vi "External Interface - Find Control Reference.vi"(0 "Control References - Top Level":refnum<vi>[](array[refnum]), 7 "Control Name":string) -> (4 "Ctl Refnum":refnum<vi>, 8 "Found":bool, 15 "error out":errorcluster)   [LabVIEW 2010]
panel:
  out "Control Names":string[](array[string])
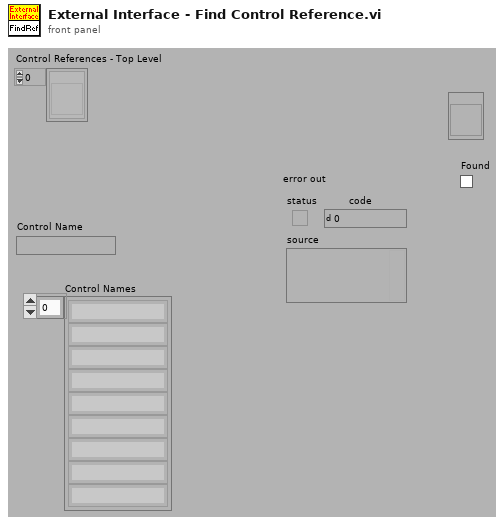
[diagram p1: front panel]
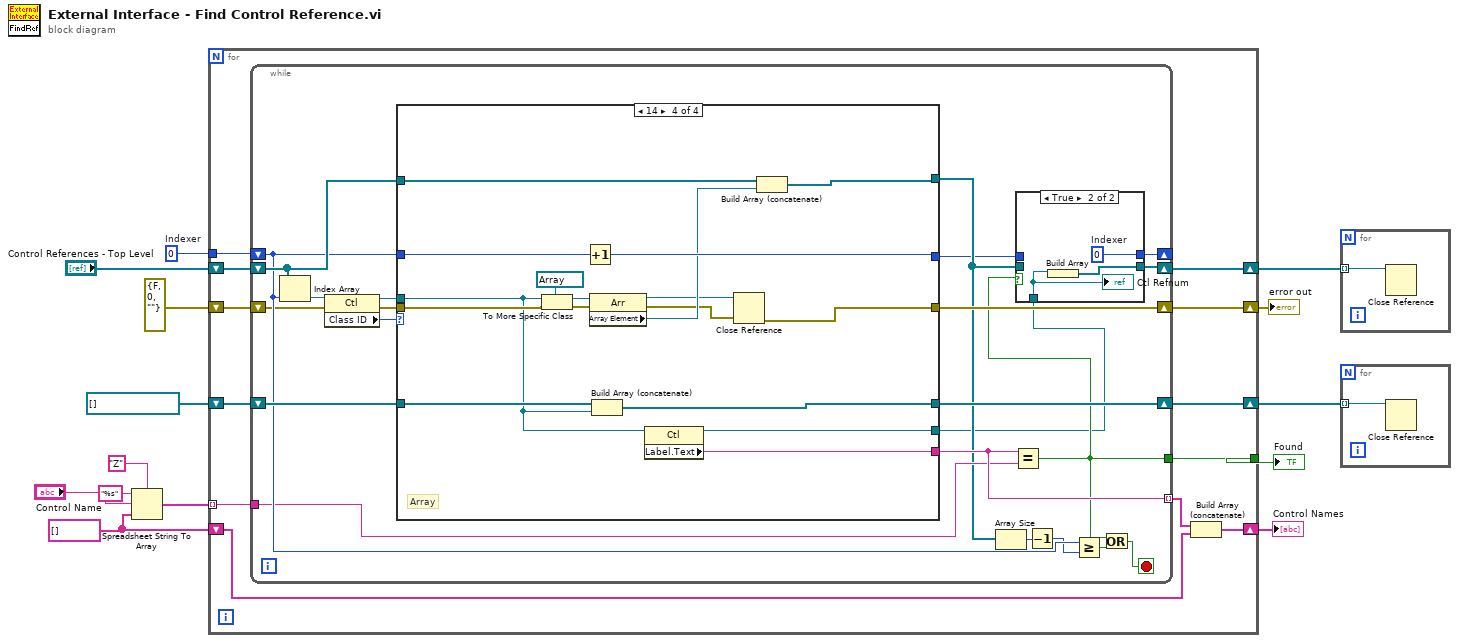
[diagram p0: block diagram]
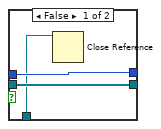
[diagram p2: hidden frame]
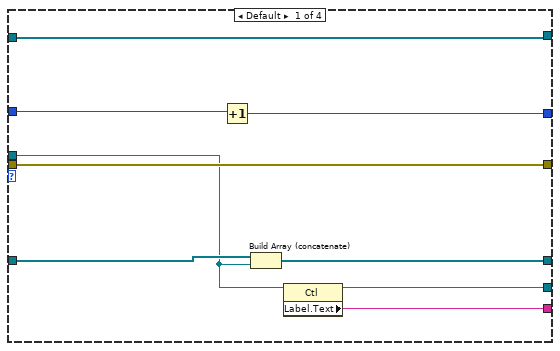
[diagram p3: hidden frame]
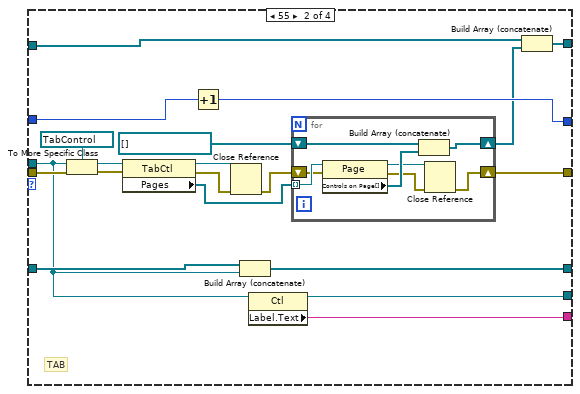
[diagram p4: hidden frame]
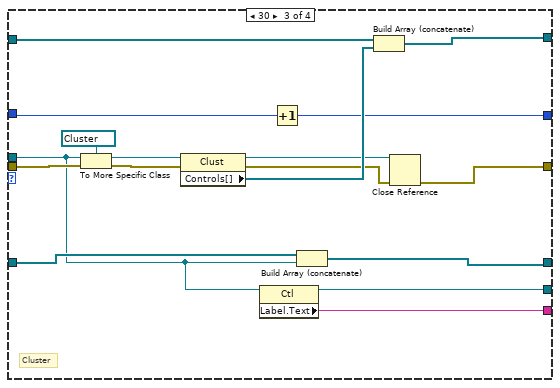
[diagram p5: hidden frame]
diagram:
  w4 = string[] []
  w13 = 0  # Indexer
  n1 = Spreadsheet String To Array(delimiter (Tab)="Ζ", format string="%s", spreadsheet string="Control Name", array type (2D Dbl)=w4) -> (array=w6:string[])
  n2 = for {
    tunnel: w13 -> [w25]
    tunnel: [w22] -> w10
    tunnel: w6 -> [w20] mode=indexing
    shift-right: [w24] -> w12
    shift-left: errorcluster {"status"=FALSE, "code"=0, "source"=""} ("error in") -> [w23]
    shift-right: [w21] -> w2
    shift-left: refnum<vi>[] [] -> [w26]
    shift-right: [w19] -> w1
    shift-left: "Control References - Top Level" -> [w18]
    shift-right: [w15] -> w3
    shift-left: w4 -> [w16]
    n3 = while {
      shift-right: [w46] -> w21
      shift-left: w26 -> [w47]
      shift-right: [w31] -> w19
      shift-left: w18 -> [w44]
      shift-right: [w30] -> _
      shift-left: w25 -> [w42]
      shift-right: [w40] -> w24
      shift-left: w23 -> [w41]
      tunnel: [w28] -> w22
      tunnel: [w34] -> w17 mode=indexing
      tunnel: w20 -> [w33]
      stop <- w35 stop-if-true
      n4 = Index Array(array=w44, index=w42) -> (element=w45:refnum<vi>)
      n5 = property class="Ctl"(reference=w45, error in=w41) -> (reference out=w48:refnum<vi>, error out=w39:errorcluster, "Class ID"=w37:u32)
      n6 = case shown="14" w37 {
        tunnel: w48 -> [w57 w70 w97 w114]
        tunnel: w47 -> [w58 w71 w101 w116]
        tunnel: [w63 w77 w102 w115] -> w46
        tunnel: [w62 w81 w108 w122] -> w32
        tunnel: w44 -> [w62 w79 w99 w123]
        tunnel: w42 -> [w61 w76 w100 w121]
        tunnel: [w60 w80 w98 w124] -> w29
        tunnel: w39 -> [w59 w74 w106 w119]
        tunnel: [w59 w72 w92 w109] -> w40
        tunnel: [w56 w69 w96 w113] -> w34
        tunnel: [w55 w68 w95 w112] -> w27
        frame Default {
          n7 = Increment(x=w61) -> (x+1=w60:i32)
          n8 = Build Array (concatenate)(w58, w57) -> (w63:refnum<vi>[])
          n9 = property class="Ctl"(reference=w57) -> (reference out=w55:refnum<vi>, "Label.Text"=w56:string)  [unwired: 1 in, 1 out]
        }
        frame 55 {
          # "TAB"
          n10 = To More Specific Class(target class=refnum<vi> refnum ("TabCtl Refnum"), reference=w70, error in=w74) -> (specific class reference=w83:refnum<vi>, error out=w73:errorcluster)
          n11 = property class="TabCtl"(reference=w83, error in=w73) -> (reference out=w66:refnum<vi>, error out=w65:errorcluster, "Pages"=w67:refnum<vi>[])
          n12 = Increment(x=w76) -> (x+1=w80:i32)
          n13 = Close Reference(reference=w66, error in (no error)=w65) -> (error out=w64:errorcluster)
          n14 = Build Array (concatenate)(w71, w70) -> (w77:refnum<vi>[])
          n15 = property class="Ctl"(reference=w70) -> (reference out=w68:refnum<vi>, "Label.Text"=w69:string)  [unwired: 1 in, 1 out]
          n16 = for {
            tunnel: w67 -> [w91] mode=indexing
            shift-right: [w89] -> w78
            shift-left: refnum<vi>[] [] -> [w90]
            shift-right: [w84] -> w72
            shift-left: w64 -> [w88]
            n17 = property class="Page"(reference=w91, error in=w88) -> (reference out=w86:refnum<vi>, error out=w85:errorcluster, "Controls on Page[]"=w87:refnum<vi>[])
            n18 = Build Array (concatenate)(w90, w87) -> (w89:refnum<vi>[])
            n19 = Close Reference(reference=w86, error in (no error)=w85) -> (error out=w84:errorcluster)
          }
          n20 = Build Array (concatenate)(w79, w78) -> (w81:refnum<vi>[])
        }
        frame 30 {
          # "Cluster"
          n21 = To More Specific Class(target class=refnum<vi> refnum ("Clust Refnum"), reference=w97, error in=w106) -> (specific class reference=w103:refnum<vi>, error out=w105:errorcluster)
          n22 = property class="Clust"(reference=w103, error in=w105) -> (reference out=w94:refnum<vi>, error out=w93:errorcluster, "Controls[]"=w104:refnum<vi>[])
          n23 = property class="Ctl"(reference=w97) -> (reference out=w95:refnum<vi>, "Label.Text"=w96:string)  [unwired: 1 in, 1 out]
          n24 = Increment(x=w100) -> (x+1=w98:i32)
          n25 = Build Array (concatenate)(w101, w97) -> (w102:refnum<vi>[])
          n26 = Build Array (concatenate)(w99, w104) -> (w108:refnum<vi>[])
          n27 = Close Reference(reference=w94, error in (no error)=w93) -> (error out=w92:errorcluster)
        }
        frame 14 {
          # "Array"
          n28 = To More Specific Class(target class=refnum<vi> refnum ("Array Refnum"), reference=w114, error in=w119) -> (specific class reference=w125:refnum<vi>, error out=w118:errorcluster)
          n29 = Increment(x=w121) -> (x+1=w124:i32)
          n30 = property class="Arr"(reference=w125, error in=w118) -> (reference out=w111:refnum<vi>, error out=w110:errorcluster, "Array Element"=w117:refnum<vi>)
          n31 = Build Array (concatenate)(w116, w114) -> (w115:refnum<vi>[])
          n32 = property class="Ctl"(reference=w114) -> (reference out=w112:refnum<vi>, "Label.Text"=w113:string)  [unwired: 1 in, 1 out]
          n33 = Close Reference(reference=w111, error in (no error)=w110) -> (error out=w109:errorcluster)
          n34 = Build Array (concatenate)(w123, w117) -> (w122:refnum<vi>[])
        }
      }
      n35 = Array Size(array=w32) -> (size(s)=w43:i32)
      n36 = Equal?(x=w34, y=w33) -> (x = y?=w28:bool)
      n37 = case shown="True" w28 {
        tunnel: w32 -> [w51 _]
        tunnel: [w51 w53] -> w31
        tunnel: [w50 w54] -> w30
        tunnel: w29 -> [w50 _]
        tunnel: w27 -> [w49 w52]
        frame False {
          n38 = Close Reference(reference=w49) -> ()  [unwired: 1 in, 1 out]
        }
        frame True {
          w54 = 0  # Indexer
          n39 = Build Array(w52) -> (w53:refnum<vi>[])
          "Ctl Refnum" <- w52
        }
      }
      n40 = Decrement(x=w43) -> (x-1=w38:i32)
      n41 = Greater Or Equal?(x=w42, y=w38) -> (x >= y?=w36:bool)
      n42 = Or(x=w28, y=w36) -> (x .or. y?=w35:bool)
    }
    n43 = Build Array (concatenate)(w17, w16) -> (w15:string[])
  }
  "error out" <- w12
  "Found" <- w10
  "Control Names" <- w3
  n44 = for {
    tunnel: w1 -> [w126] mode=indexing
    n45 = Close Reference(reference=w126) -> ()  [unwired: 1 in, 1 out]
  }
  n46 = for {
    tunnel: w2 -> [w127] mode=indexing
    n47 = Close Reference(reference=w127) -> ()  [unwired: 1 in, 1 out]
  }
